vi "Cancel State Machine.vi"(0 "What to Cancel":enum16{"Pickup", "Load"}(ring)) -> ()   [LabVIEW 2013]
uses:
  typedefs/fg_typedef.ctl
  typedefs/subStates.ctl
  typedefs/singleUseSubstate.ctl
panel:
  # "A State Machine to Handle Canceling Last Given Command"
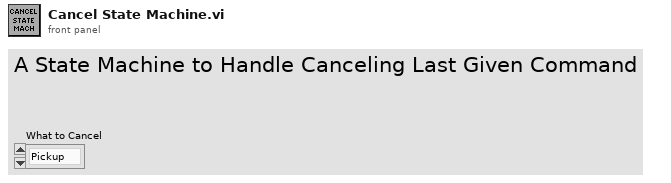
[diagram p1: front panel]
types:
  T1 = typedef "fg_typedef.ctl" = enum16{"Get", "Set"}
  T2 = typedef "subStates.ctl" = enum16{"null", "wait", "driver control", "auto", "manual override", "hold position", "rotate", "pickup", "pass", "load", "goto shoot", "shoot high goal", "shoot low goal", "cancel arm", "cancel shooter", "end"}
  T3 = typedef "singleUseSubstate.ctl" = enum16{"null", "wait", "shift high", "shift low", "cock shooter", "retract shooter", "latch", "unlatch"}
  T4 = typedef "WPI_DigitalInputDevRef.ctl" = cluster{"DevStatus":errorcluster, "DIO Channel":T5, "Digital Module":T6}
  T5 = typedef "FPGA_DIOChannel.ctl" = enum8{"DIO 1", "DIO 2", "DIO 3", "DIO 4", "DIO 5", "DIO 6", "DIO 7", "DIO 8", "DIO 9", "DIO 10", "DIO 11", "DIO 12", "DIO 13", "DIO 14", "Invalid"}
  T6 = typedef "FPGA_TypedefDigitalModule.ctl" = enum16{"Digital Module 1", "Digital Module 2"}
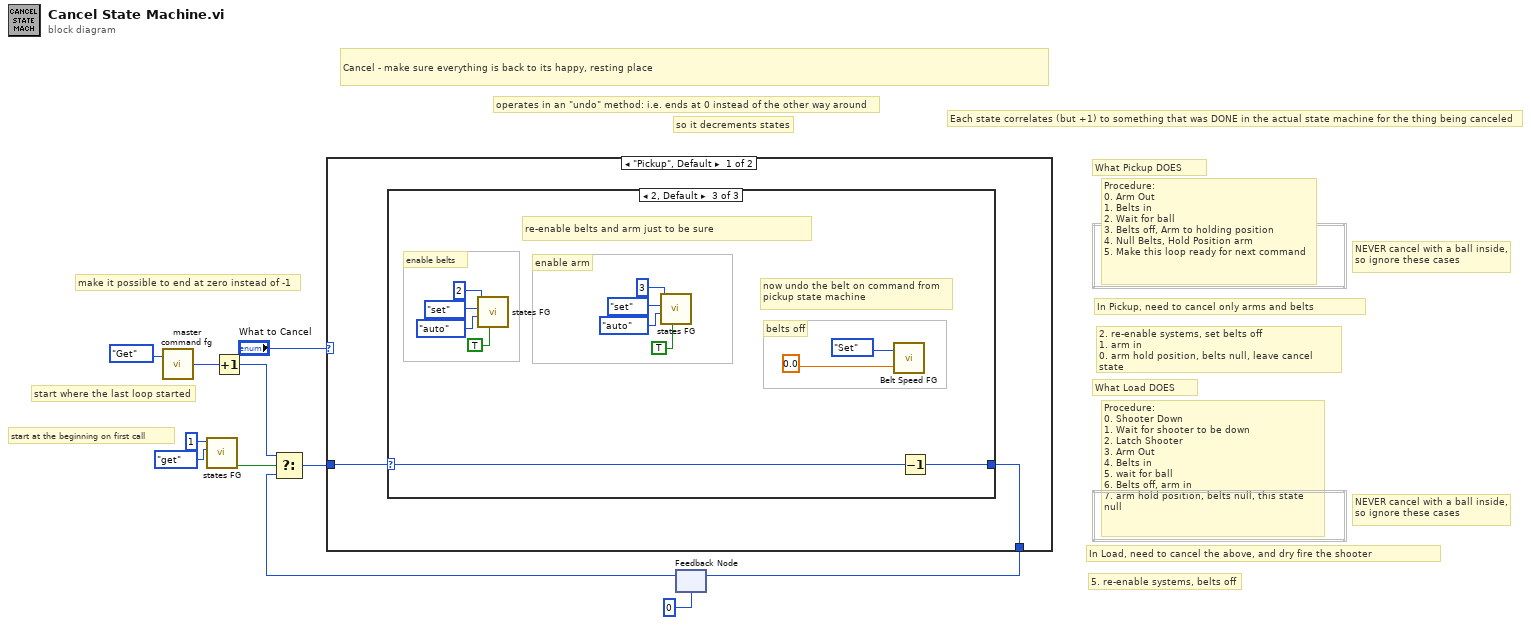
[diagram p0: block diagram]
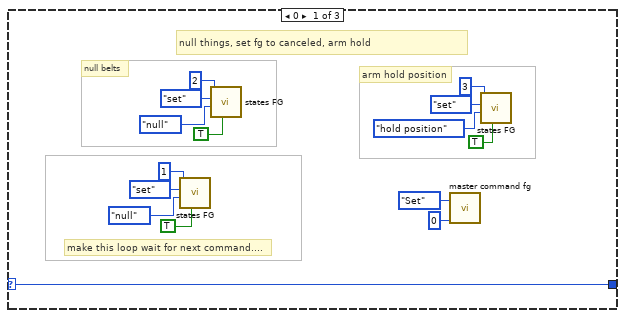
[diagram p2: hidden frame]
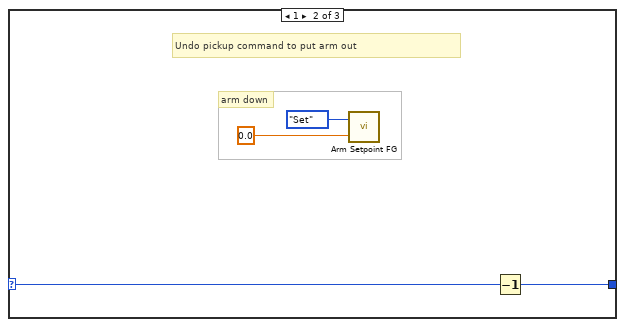
[diagram p3: hidden frame]
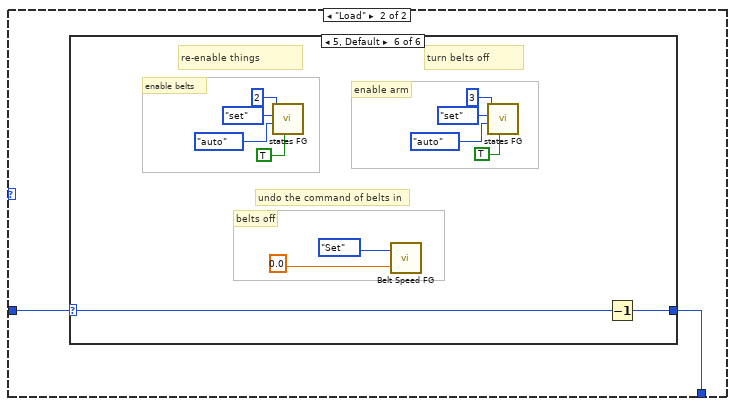
[diagram p4: hidden frame]
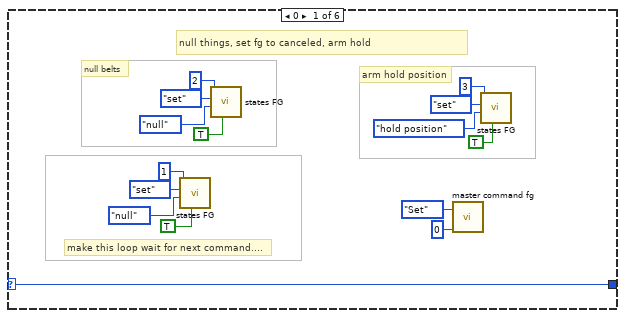
[diagram p5: hidden frame]
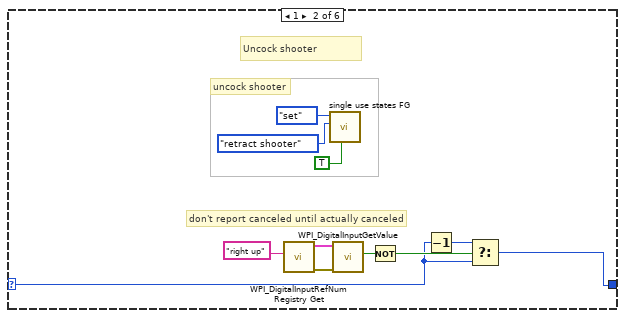
[diagram p6: hidden frame]
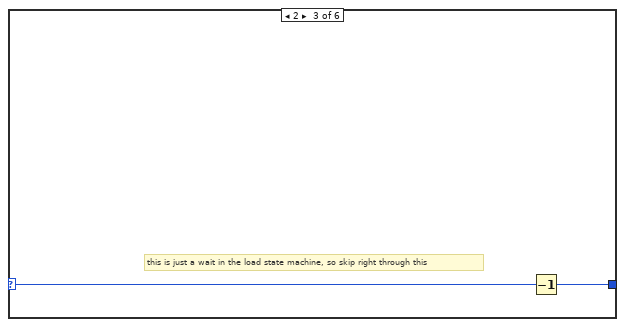
[diagram p7: hidden frame]
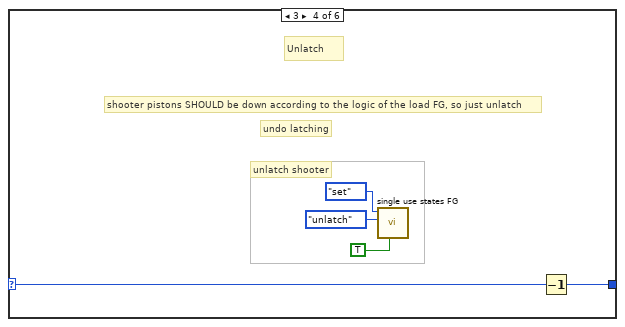
[diagram p8: hidden frame]
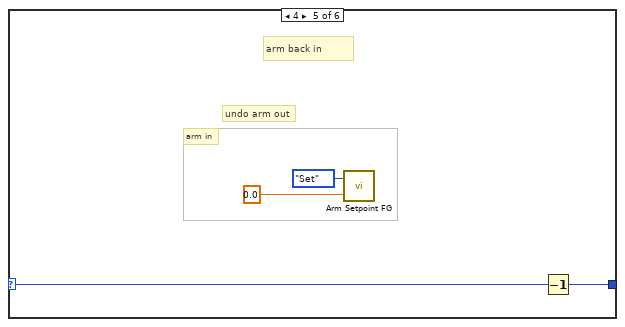
[diagram p9: hidden frame]
diagram:
  # "NEVER cancel with a ball inside,\nso ignore these cases"
  # "Procedure: \n0. Shooter Down\n1. Wait for shooter to be down\n2. Latch Shooter\n3. Arm Out\n4. Belts in\n5. wait for ball\n6. Belts off, arm in\n7. arm hold position, belts null, this state null"
  # "What Load DOES"
  # "NEVER cancel with a ball inside,\nso ignore these cases"
  # "so it decrements states"
  # "Procedure: \n0. Arm Out\n1. Belts in\n2. Wait for ball\n3. Belts off, Arm to holding position\n4. Null Belts, Hold Position arm\n5. Make this loop ready for next command"
  # "What Pickup DOES"
  # "make it possible to end at zero instead of -1"
  # "Each state correlates (but +1) to something that was DONE in the actual state machine for the thing being canceled"
  # "5. re-enable systems, belts off"
  # "In Load, need to cancel the above, and dry fire the shooter"
  # "operates in an \"undo\" method: i.e. ends at 0 instead of the other way around"
  # "start where the last loop started"
  # "2. re-enable systems, set belts off\n1. arm in\n0. arm hold position, belts null, leave cancel state"
  # "In Pickup, need to cancel only arms and belts"
  # "start at the beginning on first call"
  # "Cancel - make sure everything is back to its happy, resting place"
  n1 = call "master command fg.vi"("Menu"=fg_typedef."Get") -> ("Loop Progress"=w4:u8)  [unwired: 1 in]
  n2 = call "states FG.vi"("menu (get)"=enum16{"set", "get"}."get", "Loop ID"=1) -> ("first call?"=w10:bool)  [unwired: 6 in, 3 out]
  n3 = Increment(x=w4) -> (x+1=w2:u8)
  n4 = feedback #1(u8 0) -> (w5:u8)
  n5 = Select(t=w2, s=w10, f=w5) -> (s? t:f=w7:u8)
  n6 = case shown="\"Pickup\", Default" "What to Cancel" {
    tunnel: w7 -> [w13 w46]
    tunnel: [w12 w45] -> w3
    frame "Pickup", Default {
      n7 = case shown="2, Default" w13 {
        selector: w13 -> [w28 w32 w34]
        tunnel: [w28 w31 w33] -> w12
        frame 0 {
          # "null things, set fg to canceled, arm hold"
          # "make this loop wait for next command...."
          # "arm hold position"
          # "null belts"
          n8 = call "states FG.vi"("exit in"=TRUE, "subState in"=subStates."null", "menu (get)"=enum16{"set", "get"}."set", "Loop ID"=1) -> ()  [unwired: 4 in, 4 out]
          n9 = call "states FG.vi"("exit in"=TRUE, "subState in"=subStates."null", "menu (get)"=enum16{"set", "get"}."set", "Loop ID"=2) -> ()  [unwired: 4 in, 4 out]
          n10 = call "master command fg.vi"("Loop Progress"=u8 0, "Menu"=fg_typedef."Set") -> ()  [unwired: 1 out]
          n11 = call "states FG.vi"("exit in"=TRUE, "subState in"=subStates."hold position", "menu (get)"=enum16{"set", "get"}."set", "Loop ID"=3) -> ()  [unwired: 4 in, 4 out]
        }
        frame 1 {
          # "arm down"
          # "Undo pickup command to put arm out"
          n12 = call "Arm Setpoint FG.vi"("Setpoint In"=0.0, "Menu"=fg_typedef."Set") -> ()  [unwired: 1 out]
          n13 = Decrement(x=w32) -> (x-1=w31:u8)
        }
        frame 2, Default {
          # "now undo the belt on command from\npickup state machine"
          # "belts off"
          # "re-enable belts and arm just to be sure"
          # "enable arm"
          # "enable belts"
          n14 = call "states FG.vi"("exit in"=TRUE, "subState in"=subStates."auto", "menu (get)"=enum16{"set", "get"}."set", "Loop ID"=2) -> ()  [unwired: 4 in, 4 out]
          n15 = call "states FG.vi"("exit in"=TRUE, "subState in"=subStates."auto", "menu (get)"=enum16{"set", "get"}."set", "Loop ID"=3) -> ()  [unwired: 4 in, 4 out]
          n16 = call "Belt Speed FG.vi"("Speed In"=0.0 ("Setpoint In"), "Menu"=fg_typedef."Set") -> ()  [unwired: 1 out]
          n17 = Decrement(x=w34) -> (x-1=w33:u8)
        }
      }
    }
    frame "Load" {
      n18 = case shown="5, Default" w46 {
        selector: w46 -> [w61 w63 w74 w76 w81 w85]
        tunnel: [w61 w62 w73 w75 w80 w84] -> w45
        frame 0 {
          # "null things, set fg to canceled, arm hold"
          # "make this loop wait for next command...."
          # "arm hold position"
          # "null belts"
          n19 = call "states FG.vi"("exit in"=TRUE, "subState in"=subStates."null", "menu (get)"=enum16{"set", "get"}."set", "Loop ID"=1) -> ()  [unwired: 4 in, 4 out]
          n20 = call "states FG.vi"("exit in"=TRUE, "subState in"=subStates."null", "menu (get)"=enum16{"set", "get"}."set", "Loop ID"=2) -> ()  [unwired: 4 in, 4 out]
          n21 = call "master command fg.vi"("Loop Progress"=u8 0, "Menu"=fg_typedef."Set") -> ()  [unwired: 1 out]
          n22 = call "states FG.vi"("exit in"=TRUE, "subState in"=subStates."hold position", "menu (get)"=enum16{"set", "get"}."set", "Loop ID"=3) -> ()  [unwired: 4 in, 4 out]
        }
        frame 1 {
          # "don't report canceled until actually canceled"
          # "uncock shooter"
          # "Uncock shooter"
          n23 = call <vilib>:"WPI_DigitalInputRefNum Registry Get.vi"("refnum name"="right up") -> ("error out"=w65:errorcluster, "DigitalInputDevRef"=w66:T4)  [unwired: 9 in]
          n24 = call "single use states FG.vi"("exit in"=TRUE, "substate"=singleUseSubstate."retract shooter", "menu (get)"=enum16{"set", "get"}."set") -> ()  [unwired: 5 in, 4 out]
          n25 = call <vilib>:"WPI_DigitalInputGetValue.vi"("error in (no error)"=w65, "DigitalInputDevRef"=w66) -> ("Value"=w67:bool)  [unwired: 7 in, 2 out]
          n26 = Not(x=w67) -> (.not. x?=w69:bool)
          n27 = Decrement(x=w63) -> (x-1=w68:u8)
          n28 = Select(t=w68, s=w69, f=w63) -> (s? t:f=w62:u8)
        }
        frame 2 {
          # "this is just a wait in the load state machine, so skip right through this"
          n29 = Decrement(x=w74) -> (x-1=w73:u8)
        }
        frame 3 {
          # "unlatch shooter"
          # "undo latching"
          # "Unlatch"
          # "shooter pistons SHOULD be down according to the logic of the load FG, so just unlatch"
          n30 = call "single use states FG.vi"("exit in"=TRUE, "substate"=singleUseSubstate."unlatch", "menu (get)"=enum16{"set", "get"}."set") -> ()  [unwired: 5 in, 4 out]
          n31 = Decrement(x=w76) -> (x-1=w75:u8)
        }
        frame 4 {
          # "undo arm out"
          # "arm back in"
          # "arm in"
          n32 = call "Arm Setpoint FG.vi"("Setpoint In"=0.0, "Menu"=fg_typedef."Set") -> ()  [unwired: 1 out]
          n33 = Decrement(x=w81) -> (x-1=w80:u8)
        }
        frame 5, Default {
          # "re-enable things"
          # "turn belts off"
          # "undo the command of belts in"
          # "belts off"
          # "enable arm"
          # "enable belts"
          n34 = call "states FG.vi"("exit in"=TRUE, "subState in"=subStates."auto", "menu (get)"=enum16{"set", "get"}."set", "Loop ID"=2) -> ()  [unwired: 4 in, 4 out]
          n35 = call "Belt Speed FG.vi"("Speed In"=0.0 ("Setpoint In"), "Menu"=fg_typedef."Set") -> ()  [unwired: 1 out]
          n36 = call "states FG.vi"("exit in"=TRUE, "subState in"=subStates."auto", "menu (get)"=enum16{"set", "get"}."set", "Loop ID"=3) -> ()  [unwired: 4 in, 4 out]
          n37 = Decrement(x=w85) -> (x-1=w84:u8)
        }
      }
    }
  }
  n38 = feedback-in #1(w3) -> ()
